vi "Read RetentionPolicy.vi"(11 "DataPoint in":refnum<class "DataPoint.lvclass">) -> (2 "RetentionPolicy.lvclass":refnum<class "RetentionPolicy.lvclass">, 3 "DataPoint out":refnum<class "DataPoint.lvclass">)   [LabVIEW 2018, in "InfluxDB Client.lvlib" / "DataPoint.lvclass"]
uses:
  DataPoint.lvclass
  RetentionPolicy/RetentionPolicy.lvclass
  DataPoint.lvclass/DataPoint.ctl
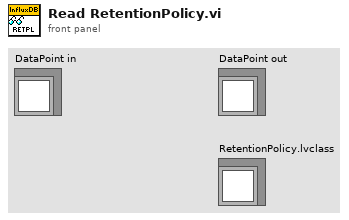
[diagram p1: front panel]
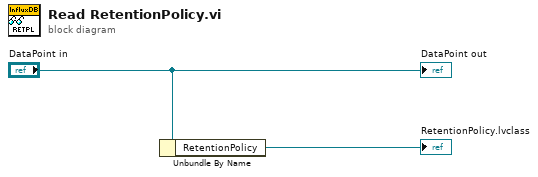
[diagram p0: block diagram]
diagram:
  n1 = Unbundle By Name("DataPoint in") -> ("RetentionPolicy"=→"RetentionPolicy.lvclass":refnum<class "RetentionPolicy.lvclass">)
  "DataPoint out" <- "DataPoint in"
